vi "FGVQ.vi"(7 "State":T1, 8 "Error In":errorcluster) -> (0 "Error Out":errorcluster, 3 "queue out":refnum<queue>)   [LabVIEW 2017, in "Controller.lvlib"]
uses:
  Controller.lvlib
  States_FGVQ.ctl
  MessageData.ctl
  States_Module.ctl
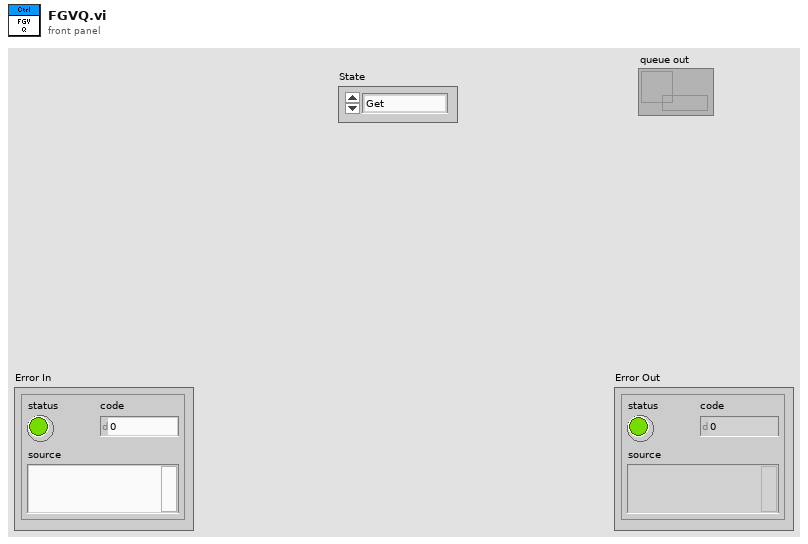
[diagram p1: front panel]
types:
  T1 = typedef "Controller.lvlib/States_FGVQ.ctl" = enum16{"Get", "Shutdown", "Initialize"}
  T2 = typedef "Controller.lvlib/MessageData.ctl" = cluster{"State":T3, "Payload":variant, "WaitOnReply":bool, "ReplyNotif":refnum<notifier>}
  T3 = typedef "Controller.lvlib/States_Module.ctl" = enum16{"DoSomething", "Shutdown", "Initialize"}
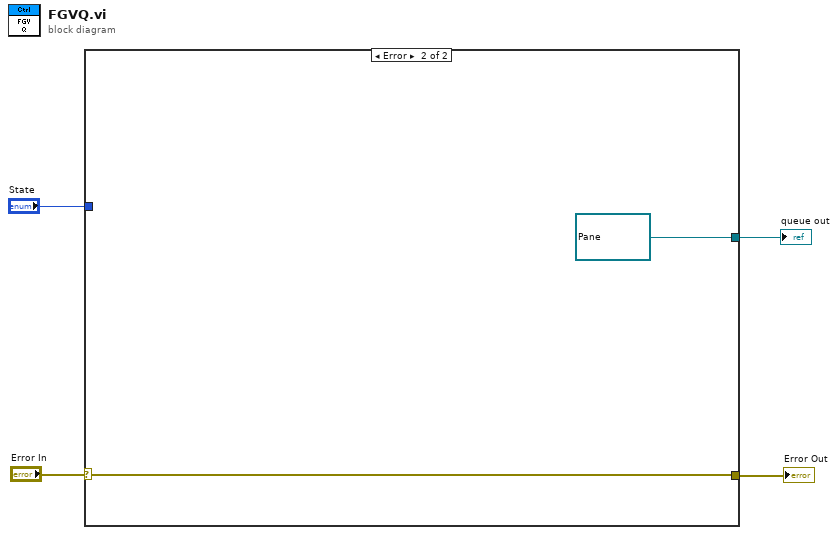
[diagram p0: block diagram]
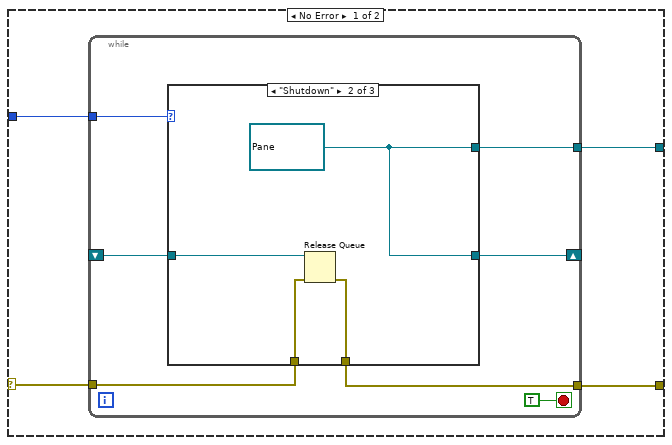
[diagram p2: hidden frame]
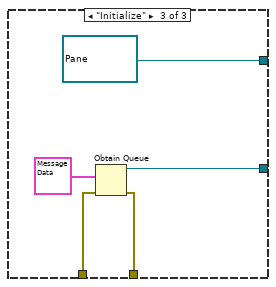
[diagram p4: hidden frame]
diagram:
  n1 = case shown="Error" "Error In" {
    selector: "Error In" -> [w8 w28]
    tunnel: "State" -> [w7 _]
    tunnel: [w6 w28] -> w2
    tunnel: [w5 refnum<queue> refnum ("queue out")] -> w1
    frame No Error {
      n2 = while {
        tunnel: w8 -> [w13]
        tunnel: w7 -> [w14]
        tunnel: [w12] -> w6
        shift-right: [w11] -> _
        shift-left: _ -> [w10]
        tunnel: [w9] -> w5
        stop <- TRUE stop-if-true
        n3 = case shown="\"Shutdown\"" w14 {
          tunnel: w13 -> [w16 w20 w25]
          tunnel: [w16 w19 w24] -> w12
          tunnel: [w17 w18 w23] -> w11
          tunnel: w10 -> [w17 w21 _]
          tunnel: [w17 w18 refnum<queue> refnum ("queue out")] -> w9
          frame "Get", Default {
          }
          frame "Shutdown" {
            w18 = refnum<queue> refnum ("queue out")
            n4 = Release Queue(queue=w21, error in (no error)=w20) -> (error out=w19:errorcluster)  [unwired: 1 in, 2 out]
          }
          frame "Initialize" {
            n5 = Obtain Queue(element data type=T2 {"State"=enum."DoSomething", "Payload"=variant, "WaitOnReply"=TRUE, "ReplyNotif"=refnum}, error in (no error)=w25) -> (queue out=w23:refnum<queue>, error out=w24:errorcluster)  [unwired: 3 in, 1 out]
          }
        }
      }
    }
    frame Error {
    }
  }
  "Error Out" <- w2
  "queue out" <- w1
